vi "5.0.1_LL_Restriction.vi"(6 "Data in":T1, 8 "error in (no error)":errorcluster, 9 "AllControls In":T2, 10 "?":T3, 11 "Message Queue out":T4) -> (0 "error out":errorcluster, 1 "Flow":string, 2 "Data":T3, 3 "Message Queue Out":T4, 4 "Data out":T1)   [LabVIEW 2017]
uses:
  Depends/AMC/subVIs/TypeDefs/amc_Message Queue.ctl
  Depends/AMC/subVIs/TypeDefs/amc_Message.ctl
  Depends/Tools/Keyed Array/Tools_KeyedArray KeyedArray.ctl
  Ctrls/Data.ctl
  Ctrls/AllControls.ctl
  Ctrls/CSV_Data.ctl
  Ctrls/AlarmIndex.ctl
  DIPC 692 Daemon API/typdef/get_parameter.ctl
  DIPC 692 Daemon API/typdef/task_detect_test_point.ctl
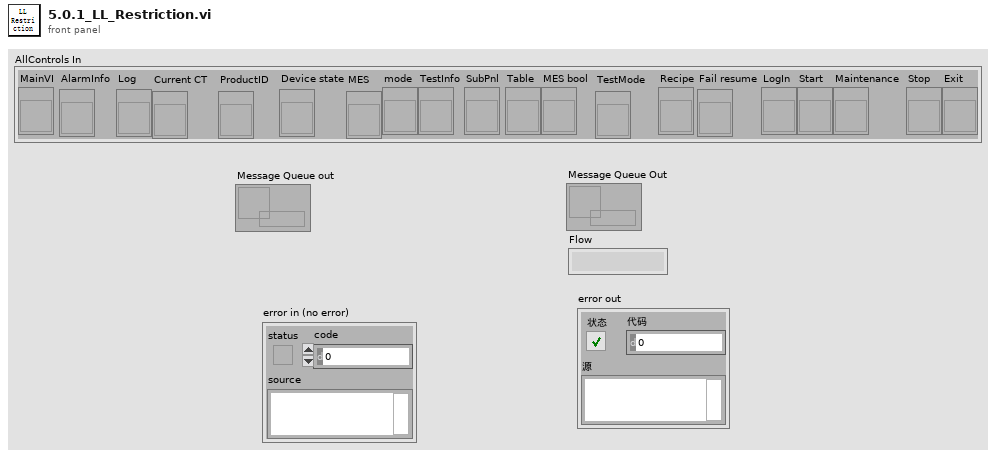
[diagram p1: front panel]
types:
  T1 = typedef "CSV_Data.ctl" = cluster{"Initialisation":cluster{"LMT - Connect UUT (con COM)":string, "LMT - Software Version (rrel)":string, "LMT - Write SKU file (wskuc)":string, "LMT - SKU file name":string, "Connect UUT DDM":string, "Read DDM EOL Timestamp - Mode":string, "Read DDM EOL Timestamp - Timestamp":string, "Read DDM EOL Timestamp - Rig ID":string, "Read DDM EOL Timestamp - Passmark ID":string, "Read DDM EOL Timestamp - Passmark Rev":string, "Software Version before flashing":string, "Read Hardware Serial":string, "UUT DDM SN":string, "Compare DDM SN with MES SN":string, "Backup PCBA Calibration EEPROM Response - CAL":string, "Flash Firmware Version":string, "Check SW Version":string, "Read DDM SW Version after flashing":string, "Set SKU Config":string, "Ready Status":string, "Set Device Mode to EOL":string, "DDM Parameter - Voltage":string, "DDM Parameter - Current":string, "DDM Parameter - Power":string, "DDM Parameter - Speed":string, "DDM Parameter - Pressure":string, "Tester Parameter - Voltage":string, "Tester Parameter - Current":string, "Tester Parameter - Power":string, "Tester Parameter - Ambient Pressure":string, "Tester Parameter - Ambient Temperature":string, "Calculated Parameter - DDM Pressure Corrected":string, "Calculated Parameter - DDM Real Power":string, "Calculated Parameter - Delta V":string}, "BEMF_Calibration":cluster{"Calibration Result - eol_cold_bemf_temp":string, "DDM Ambient Temp":string, "Restriction Plate Diameter":string, "Calibration Result - eol_bemf_mp_cold_coef_a":string, "Calibration Result - eol_bemf_mp_cold_coef_b":string, "Calibration Result - eol_bemf_mp_cold_coef_c":string, "Calibration Result - eol_bemf_lsi_cold_ref_coeffs":string, "Get - Calibration Result - eol_bemf_lsi_speed":string, "Get - Calibration Result - eol_bemf_lsi_integral_0":string, "Calibration Result - eol_bemf_lsi_integral_1":string, "Get - Calibration Result - eol_bemf_lsi_integral_2":string, "Get - Calibration Result - eol_cold_bemf":string, "Get - Calibration Result - eol_cold_bemf_fisf":string, "Finalise Calibration":string, "Compare -Calibration Result - eol_cold_bemf":string, "Compare -Calibration Result - eol_cold_bemf_fisf":string}, "ECO":cluster{"Reset Power Tune":string, "Reset BEMF FISF Calibration":string, "Restriction Plate Diameter":string, "ECO - Stabilisation Time":string, "ECO - DDM Parameter - Voltage":string, "ECO - DDM Parameter - Current":string, "ECO - DDM Parameter - Power":string, "ECO - DDM Parameter - Measured Power":string, "ECO - DDM Parameter - Speed":string, "ECO - DDM Parameter - Pressure":string, "ECO - Tester Parameter - Voltage":string, "ECO - Tester Parameter - Current":string, "ECO - Tester Parameter - Power":string, "ECO - Tester Parameter - Ambient Pressure":string, "ECO - Tester Parameter - Ambient Temperature":string, "ECO - Tester Parameter - Ambient Humidity":string, "ECO - Calculated Parameter - DDM Pressure Corrected":string, "ECO - Calculated Parameter - DDM Real Power":string, "ECO - Calculated Parameter - Delta V":string, "ECO - Calculated Parameter - Flowrate":string, "ECO - Calculated Parameter - Airwatt":string, "ECO - Formula":string, "PT ECO - Power Tune Mode Status":string}, "BOOST":cluster{"Restriction Plate Diameter":string, "BOOST - Stabilisation Time":string, "BOOST - DDM Parameter - Voltage":string, "BOOST - DDM Parameter - Current":string, "BOOST - DDM Parameter - Power":string, "BOOST - DDM Parameter - Measured Power":string, "BOOST - DDM Parameter - Speed":string, "BOOST - DDM Parameter - Pressure":string, "BOOST - Tester Parameter - Voltage":string, "BOOST - Tester Parameter - Current":string, "BOOST - Tester Parameter - Power":string, "BOOST - Tester Parameter - Ambient Pressure":string, "BOOST - Tester Parameter - Ambient Temperature":string, "BOOST - Tester Parameter - Ambient Humidity":string, "BOOST - Calculated Parameter - DDM Pressure Corrected":string, "BOOST - Calculated Parameter - DDM Real Power":string, "BOOST - Calculated Parameter - Delta V":string, "BOOST - Calculated Parameter - Flowrate":string, "BOOST - Calculated Parameter - Airwatt":string, "BOOST - Get AM Presence":string, "Air Muscle Turn Off Status":string, "BOOST - Air Muscle Calculated Parameter - Airwatt B":string, "BOOST - Air Muscle Calculate Airwatt Delta":string, "PT BOOST - Power Tune Mode Status":string, "Finalise Calibration":string, "ECO - Get AW Calibration value":string, "BOOST - Get AW Calibration value":string}, "MAX":cluster{"Restriction Plate Diameter":string, "MAX - Stabilisation Time":string, "Get Average Delta Tmag (LSIdelta_FISFdelta_LSItmag_FISFtmag_IIRtmag)":string, "Get Average Delta Tmag FISF":string, "MAX - DDM Parameter - Voltage":string, "MAX - DDM Parameter - Current":string, "MAX - DDM Parameter - Power":string, "MAX - DDM Parameter - Measured Power":string, "MAX - DDM Parameter - Speed":string, "MAX - DDM Parameter - Pressure":string, "MAX - Tester Parameter - Voltage":string, "MAX - Tester Parameter - Current":string, "MAX - Tester Parameter - Power":string, "MAX - Tester Parameter - Ambient Pressure":string, "MAX - Tester Parameter - Ambient Temperature":string, "MAX - Tester Parameter - Ambient Humidity":string, "MAX - Calculated Parameter - DDM Pressure Corrected":string, "MAX - Calculated Parameter - DDM Real Power":string, "MAX - Calculated Parameter - Delta V":string, "MAX - Calculated Parameter - Flowrate":string, "MAX - Calculated Parameter - Airwatt":string, "MAX_FISF_Check_Average_Delta_Tmag":string, "MAX - FISF - BEMF Finetune Result":string, "MAX tune - Delta P1":string, "MAX tune - Calculated Parameter - Airwatt":string, "Calculate Delta Airwatts - MAX finetune - Delta P2":string, "MAX finetune - DDM Parameter - Voltage":string, "MAX finetune - DDM Parameter - Current":string, "MAX finetune - DDM Parameter - Power":string, "MAX finetune - DDM Parameter - Measured Power":string, "MAX finetune - DDM Parameter - Speed":string, "MAX finetune - DDM Parameter - Pressure":string, "MAX finetune - Tester Parameter - Voltage":string, "MAX finetune - Tester Parameter - Current":string, "MAX finetune - Tester Parameter - Power":string, "MAX finetune - Tester Parameter - Ambient Pressure":string, "MAX finetune - Tester Parameter - Ambient Temperature":string, "MAX finetune - Tester Parameter - Ambient Humidity":string, "MAX finetune - Calculated Parameter - DDM Pressure Corrected":string, "MAX finetune - Calculated Parameter - DDM Real Power":string, "MAX finetune - Calculated Parameter - Delta V":string, "MAX finetune - Calculated Parameter - Flowrate":string, "MAX finetune - Calculated Parameter - Airwatt":string, "Check Derate Result":string, "Delta Tmag FISF":string, "Get Hot BEMF Result":string, "Calculate delta Pressure":string, "Finalise Calibration":string, "Calculate & Check Delta BEMF":string, "Delta P Airwatts Value":string}, "LL":cluster{"DDM Ambient Temp":string, "Restriction Plate Diameter":string, "LL - DDM Parameter - Voltage":string, "LL - DDM Parameter - Current":string, "LL - DDM Parameter - Power":string, "LL - DDM Parameter - Measured Power":string, "LL - DDM Parameter - Speed":string, "LL - DDM Parameter - Pressure":string, "LL - Tester Parameter - Voltage":string, "LL - Tester Parameter - Current":string, "LL - Tester Parameter - Power":string, "LL - DDM Real Power":string, "LL - Calibrate Task Detect LL":string}, "HL":cluster{"HL - DDM Parameter - Voltage":string, "HL - DDM Parameter - Current":string, "HL - DDM Parameter - Power":string, "HL - DDM Parameter - Measured Power":string, "HL - DDM Parameter - Speed":string, "HL - DDM Parameter - Pressure":string, "HL - Tester Parameter - Voltage":string, "HL - Tester Parameter - Current":string, "HL - Tester Parameter - Power":string, "HL - DDM Real Power":string, "HL - Calibrate Task Detect HL":string}, "LH":cluster{"Restriction Plate Diameter":string, "LH - DDM Parameter - Voltage":string, "LH - DDM Parameter - Current":string, "LH - DDM Parameter - Power":string, "LH - DDM Parameter - Measured Power":string, "LH - DDM Parameter - Speed":string, "LH - DDM Parameter - Pressure":string, "LH - Tester Parameter - Voltage":string, "LH - Tester Parameter - Current":string, "LH - Tester Parameter - Power":string, "LH - DDM Real Power":string, "LH - Calibrate Task Detect LH":string}, "HH":cluster{"HH - DDM Parameter - Voltage":string, "HH - DDM Parameter - Current":string, "HH - DDM Parameter - Power":string, "HH - DDM Parameter - Measured Power":string, "HH - DDM Parameter - Speed":string, "HH - DDM Parameter - Pressure":string, "HH - Tester Parameter - Voltage":string, "HH - Tester Parameter - Current":string, "HH - Tester Parameter - Power":string, "HH - DDM Real Power":string, "HH - Calibrate Task Detect HH":string}, "Inlet Blockage Calibration":cluster{"Inlet Blockage Calibration - DDM Parameter - Voltage":string, "Inlet Blockage Calibration - DDM Parameter - Current":string, "Inlet Blockage Calibration - DDM Parameter - Power":string, "Inlet Blockage Calibration - DDM Parameter - Measured Power":string, "Inlet Blockage Calibration - DDM Parameter - Speed":string, "Inlet Blockage Calibration - DDM Parameter - Pressure":string, "Inlet Blockage Calibration - Tester Parameter - Voltage":string, "Inlet Blockage Calibration - Tester Parameter - Current":string, "Inlet Blockage Calibration - Tester Parameter - Power":string, "Inlet Blockage Calibration - DDM Real Power":string, "Calibration Inlet Blockage_E":string, "Finalise Calibration":string, "Get Task Detect LL":string, "Get Task Detect HL":string, "Get Task Detect LH":string, "Get Task Detect HH":string, "Calibration Inlet Blockage":string, "Calibration eol cold bemf temp":string}, "GOOD":cluster{"GOOD UNIT - Clear EEPROM Error Log":string, "GOOD UNIT - Write Product Timestamp - Mode":string, "GOOD UNIT - Write Product Timestamp - Timestamp":string, "GOOD UNIT - Write Product Timestamp - Rig ID":string, "GOOD UNIT - Write Product Timestamp - Passmark ID":string, "GOOD UNIT - Write Product Timestamp - Passmark Rev":string, "GOOD UNIT - Set Device Mode to PROD":string, "GOOD UNIT - Backup PCBA Calibration EEPROM Response":string, "GOOD UNIT - Check Security Bit":string, "GOOD UNIT - Set Calibration Lock":string, "GOOD UNIT - Get_Calibration_Lock":string, "GOOD UNIT - Disconnect UUT":string}, "NG":cluster{"NG UNIT - Read NVM Error":string, "NG UNIT - Set Device Mode to FCT":string, "NG UNIT - Backup PCBA Calibration EEPROM Response - CAL":string, "NG UNIT - Backup PCBA Calibration EEPROM Response - ERROR":string, "NG UNIT - Backup PCBA Calibration EEPROM Response - USAGE":string, "NG UNIT - Disconnect UUT":string}, "SN":string, "Table":string[][], "Count":cluster{"Total":i32, "OK":i32, "NG":i32, "Yield":dbl}, "Start Time":timestamp, "daemon reference":refnum<k5>, "CT":dbl, "Config":string[][], "OK/NG":bool, "Station ID":string, "MES DDM SN":string, "MES PCBA SN":string, "Retest":string, "Lux":string, "Initialisation_Status":cluster{"LMT - Connect UUT (con COM)":string, "LMT - Software Version (rrel)":string, "LMT - Write SKU file (wskuc)":string, "LMT - SKU file name":string, "Connect UUT DDM":string, "Read DDM EOL Timestamp - Mode":string, "Read DDM EOL Timestamp - Timestamp":string, "Read DDM EOL Timestamp - Rig ID":string, "Read DDM EOL Timestamp - Passmark ID":string, "Read DDM EOL Timestamp - Passmark Rev":string, "Software Version before flashing":string, "Read Hardware Serial":string, "UUT DDM SN":string, "Compare DDM SN with MES SN":string, "Backup PCBA Calibration EEPROM Response - CAL":string, "Flash Firmware Version":string, "Check SW Version":string, "Read DDM SW Version after flashing":string, "Set SKU Config":string, "Ready Status":string, "Set Device Mode to EOL":string, "DDM Parameter - Voltage":string, "DDM Parameter - Current":string, "DDM Parameter - Power":string, "DDM Parameter - Speed":string, "DDM Parameter - Pressure":string, "Tester Parameter - Voltage":string, "Tester Parameter - Current":string, "Tester Parameter - Power":string, "Tester Parameter - Ambient Pressure":string, "Tester Parameter - Ambient Temperature":string, "Calculated Parameter - DDM Pressure Corrected":string, "Calculated Parameter - DDM Real Power":string, "Calculated Parameter - Delta V":string}, "BEMF_Calibration_Status":cluster{"Calibration Result - eol_cold_bemf_temp":string, "DDM Ambient Temp":string, "Restriction Plate Diameter":string, "Calibration Result - eol_bemf_mp_cold_coef_a":string, "Calibration Result - eol_bemf_mp_cold_coef_b":string, "Calibration Result - eol_bemf_mp_cold_coef_c":string, "Calibration Result - eol_bemf_lsi_cold_ref_coeffs":string, "Get - Calibration Result - eol_bemf_lsi_speed":string, "Get - Calibration Result - eol_bemf_lsi_integral_0":string, "Calibration Result - eol_bemf_lsi_integral_1":string, "Get - Calibration Result - eol_bemf_lsi_integral_2":string, "Get - Calibration Result - eol_cold_bemf":string, "Get - Calibration Result - eol_cold_bemf_fisf":string, "Finalise Calibration":string, "Compare -Calibration Result - eol_cold_bemf":string, "Compare -Calibration Result - eol_cold_bemf_fisf":string}, "ECO_Status":cluster{"Reset Power Tune":string, "Reset BEMF FISF Calibration":string, "Restriction Plate Diameter":string, "ECO - Stabilisation Time":string, "ECO - DDM Parameter - Voltage":string, "ECO - DDM Parameter - Current":string, "ECO - DDM Parameter - Power":string, "ECO - DDM Parameter - Measured Power":string, "ECO - DDM Parameter - Speed":string, "ECO - DDM Parameter - Pressure":string, "ECO - Tester Parameter - Voltage":string, "ECO - Tester Parameter - Current":string, "ECO - Tester Parameter - Power":string, "ECO - Tester Parameter - Ambient Pressure":string, "ECO - Tester Parameter - Ambient Temperature":string, "ECO - Tester Parameter - Ambient Humidity":string, "ECO - Calculated Parameter - DDM Pressure Corrected":string, "ECO - Calculated Parameter - DDM Real Power":string, "ECO - Calculated Parameter - Delta V":string, "ECO - Calculated Parameter - Flowrate":string, "ECO - Calculated Parameter - Airwatt":string, "ECO - Formula":string, "PT ECO - Power Tune Mode Status":string}, "BOOST_Status":cluster{"Restriction Plate Diameter":string, "BOOST - Stabilisation Time":string, "BOOST - DDM Parameter - Voltage":string, "BOOST - DDM Parameter - Current":string, "BOOST - DDM Parameter - Power":string, "BOOST - DDM Parameter - Measured Power":string, "BOOST - DDM Parameter - Speed":string, "BOOST - DDM Parameter - Pressure":string, "BOOST - Tester Parameter - Voltage":string, "BOOST - Tester Parameter - Current":string, "BOOST - Tester Parameter - Power":string, "BOOST - Tester Parameter - Ambient Pressure":string, "BOOST - Tester Parameter - Ambient Temperature":string, "BOOST - Tester Parameter - Ambient Humidity":string, "BOOST - Calculated Parameter - DDM Pressure Corrected":string, "BOOST - Calculated Parameter - DDM Real Power":string, "BOOST - Calculated Parameter - Delta V":string, "BOOST - Calculated Parameter - Flowrate":string, "BOOST - Calculated Parameter - Airwatt":string, "BOOST - Get AM Presence":string, "Air Muscle Turn Off Status":string, "BOOST - Air Muscle Calculated Parameter - Airwatt B":string, "BOOST - Air Muscle Calculate Airwatt Delta":string, "PT BOOST - Power Tune Mode Status":string, "Finalise Calibration":string, "ECO - Get AW Calibration value":string, "BOOST - Get AW Calibration value":string}, "MAX_Status":cluster{"Restriction Plate Diameter":string, "MAX - Stabilisation Time":string, "Get Average Delta Tmag (LSIdelta_FISFdelta_LSItmag_FISFtmag_IIRtmag)":string, "Get Average Delta Tmag FISF":string, "MAX - DDM Parameter - Voltage":string, "MAX - DDM Parameter - Current":string, "MAX - DDM Parameter - Power":string, "MAX - DDM Parameter - Measured Power":string, "MAX - DDM Parameter - Speed":string, "MAX - DDM Parameter - Pressure":string, "MAX - Tester Parameter - Voltage":string, "MAX - Tester Parameter - Current":string, "MAX - Tester Parameter - Power":string, "MAX - Tester Parameter - Ambient Pressure":string, "MAX - Tester Parameter - Ambient Temperature":string, "MAX - Tester Parameter - Ambient Humidity":string, "MAX - Calculated Parameter - DDM Pressure Corrected":string, "MAX - Calculated Parameter - DDM Real Power":string, "MAX - Calculated Parameter - Delta V":string, "MAX - Calculated Parameter - Flowrate":string, "MAX - Calculated Parameter - Airwatt":string, "MAX_FISF_Check_Average_Delta_Tmag":string, "MAX - FISF - BEMF Finetune Result":string, "MAX tune - Delta P1":string, "MAX tune - Calculated Parameter - Airwatt":string, "Calculate Delta Airwatts - MAX finetune - Delta P2":string, "MAX finetune - DDM Parameter - Voltage":string, "MAX finetune - DDM Parameter - Current":string, "MAX finetune - DDM Parameter - Power":string, "MAX finetune - DDM Parameter - Measured Power":string, "MAX finetune - DDM Parameter - Speed":string, "MAX finetune - DDM Parameter - Pressure":string, "MAX finetune - Tester Parameter - Voltage":string, "MAX finetune - Tester Parameter - Current":string, "MAX finetune - Tester Parameter - Power":string, "MAX finetune - Tester Parameter - Ambient Pressure":string, "MAX finetune - Tester Parameter - Ambient Temperature":string, "MAX finetune - Tester Parameter - Ambient Humidity":string, "MAX finetune - Calculated Parameter - DDM Pressure Corrected":string, "MAX finetune - Calculated Parameter - DDM Real Power":string, "MAX finetune - Calculated Parameter - Delta V":string, "MAX finetune - Calculated Parameter - Flowrate":string, "MAX finetune - Calculated Parameter - Airwatt":string, "Check Derate Result":string, "Delta Tmag FISF":string, "Get Hot BEMF Result":string, "Calculate delta Pressure":string, "Finalise Calibration":string, "Calculate & Check Delta BEMF":string, "Delta P Airwatts Value":string}, "LL_Status":cluster{"DDM Ambient Temp":string, "Restriction Plate Diameter":string, "LL - DDM Parameter - Voltage":string, "LL - DDM Parameter - Current":string, "LL - DDM Parameter - Power":string, "LL - DDM Parameter - Measured Power":string, "LL - DDM Parameter - Speed":string, "LL - DDM Parameter - Pressure":string, "LL - Tester Parameter - Voltage":string, "LL - Tester Parameter - Current":string, "LL - Tester Parameter - Power":string, "LL - DDM Real Power":string, "LL - Calibrate Task Detect LL":string}, "HL_Status":cluster{"HL - DDM Parameter - Voltage":string, "HL - DDM Parameter - Current":string, "HL - DDM Parameter - Power":string, "HL - DDM Parameter - Measured Power":string, "HL - DDM Parameter - Speed":string, "HL - DDM Parameter - Pressure":string, "HL - Tester Parameter - Voltage":string, "HL - Tester Parameter - Current":string, "HL - Tester Parameter - Power":string, "HL - DDM Real Power":string, "HL - Calibrate Task Detect HL":string}, "LH_Status":cluster{"Restriction Plate Diameter":string, "LH - DDM Parameter - Voltage":string, "LH - DDM Parameter - Current":string, "LH - DDM Parameter - Power":string, "LH - DDM Parameter - Measured Power":string, "LH - DDM Parameter - Speed":string, "LH - DDM Parameter - Pressure":string, "LH - Tester Parameter - Voltage":string, "LH - Tester Parameter - Current":string, "LH - Tester Parameter - Power":string, "LH - DDM Real Power":string, "LH - Calibrate Task Detect LH":string}, "HH_Status":cluster{"HH - DDM Parameter - Voltage":string, "HH - DDM Parameter - Current":string, "HH - DDM Parameter - Power":string, "HH - DDM Parameter - Measured Power":string, "HH - DDM Parameter - Speed":string, "HH - DDM Parameter - Pressure":string, "HH - Tester Parameter - Voltage":string, "HH - Tester Parameter - Current":string, "HH - Tester Parameter - Power":string, "HH - DDM Real Power":string, "HH - Calibrate Task Detect HH":string}, "Inlet Blockage Calibration_Status":cluster{"Inlet Blockage Calibration - DDM Parameter - Voltage":string, "Inlet Blockage Calibration - DDM Parameter - Current":string, "Inlet Blockage Calibration - DDM Parameter - Power":string, "Inlet Blockage Calibration - DDM Parameter - Measured Power":string, "Inlet Blockage Calibration - DDM Parameter - Speed":string, "Inlet Blockage Calibration - DDM Parameter - Pressure":string, "Inlet Blockage Calibration - Tester Parameter - Voltage":string, "Inlet Blockage Calibration - Tester Parameter - Current":string, "Inlet Blockage Calibration - Tester Parameter - Power":string, "Inlet Blockage Calibration - DDM Real Power":string, "Calibration Inlet Blockage_E":string, "Finalise Calibration":string, "Get Task Detect LL":string, "Get Task Detect HL":string, "Get Task Detect LH":string, "Get Task Detect HH":string, "Calibration Inlet Blockage":string, "Calibration eol cold bemf temp":string}, "GOOD_Status":cluster{"GOOD UNIT - Clear EEPROM Error Log":string, "GOOD UNIT - Write Product Timestamp - Mode":string, "GOOD UNIT - Write Product Timestamp - Timestamp":string, "GOOD UNIT - Write Product Timestamp - Rig ID":string, "GOOD UNIT - Write Product Timestamp - Passmark ID":string, "GOOD UNIT - Write Product Timestamp - Passmark Rev":string, "GOOD UNIT - Set Device Mode to PROD":string, "GOOD UNIT - Backup PCBA Calibration EEPROM Response":string, "GOOD UNIT - Check Security Bit":string, "GOOD UNIT - Set Calibration Lock":string, "GOOD UNIT - Get_Calibration_Lock":string, "GOOD UNIT - Disconnect UUT":string}, "NG_Status":cluster{"NG UNIT - Read NVM Error":string, "NG UNIT - Set Device Mode to FCT":string, "NG UNIT - Backup PCBA Calibration EEPROM Response - CAL":string, "NG UNIT - Backup PCBA Calibration EEPROM Response - ERROR":string, "NG UNIT - Backup PCBA Calibration EEPROM Response - USAGE":string, "NG UNIT - Disconnect UUT":string}, "SKU":string, "Plate_Diameter":string, "Alarm":string}
  T2 = typedef "AllControls.ctl" = cluster{"MainVI":refnum<vi>, "AlarmInfo":refnum<vi>, "Log":refnum<vi>, "Current CT":refnum<vi>, "ProductID":refnum<vi>, "Device state":refnum<vi>, "MES":refnum<vi>, "mode":refnum<vi>, "TestInfo":refnum<vi>, "SubPnl":refnum<vi>, "Table":refnum<vi>, "MES bool":refnum<vi>, "TestMode":refnum<vi>, "Recipe":refnum<vi>, "Fail resume":refnum<vi>, "LogIn":refnum<vi>, "Start":refnum<vi>, "Maintenance":refnum<vi>, "Stop":refnum<vi>, "Exit":refnum<vi>}
  T3 = typedef "Data.ctl" = cluster{"Initialisation":cluster{"DDM_Parameter":dbl[], "DDM_Parameter_status":bool[], "Get_Tester_Parameter":dbl[], "Get_Tester_Parameter_status":bool[], "Cal_Tester_Parameter":dbl[], "Cal_Tester_Parameter_status":bool[], "sw_version_before_status":bool, "sw_version_after_status":bool, "Set_SKU_Config_With_LMT_status":bool, "FCT_timestamp_status":bool, "LMT_Connect_to_UUT_status":bool}, "BEMF_Calibration":cluster{"Read_ambient_temperature":dbl, "Calibration_Vaule":dbl[], "Calibration_Vaule _B":dbl[], "Calibration_Vaule_status":bool[], "Calibration_Vaule_B_status":bool[]}, "ECO":cluster{"DDM_Parameter":dbl[], "DDM_Parameter_status":bool[], "Get_Tester_Parameter":dbl[], "Get_Tester_Parameter_status":bool[], "Cal_Tester_Parameter":dbl[], "Cal_Tester_Parameter_status":bool[], "DDM_Parameter_after_power_tune":dbl[], "Get_Tester_Parameter_after_power_tune":dbl[], "Cal_Tester_Parameter_after_power_tune":dbl[], "Cal_Tester_Parameter_after_power_tune_status":bool[], "Delta_P":dbl}, "BOOST":cluster{"DDM_Parameter":dbl[], "DDM_Parameter_status":bool[], "Get_Tester_Parameter":dbl[], "Get_Tester_Parameter_status":bool[], "Cal_Tester_Parameter":dbl[], "Cal_Tester_Parameter_status":bool[], "DDM_Parameter_after_power_tune":dbl[], "Get_Tester_Parameter_after_power_tune":dbl[], "Cal_Tester_Parameter_after_power_tune":dbl[], "Cal_Tester_Parameter_after_power_tune_status":bool[], "airwatts_am_off":dbl, "AW_Delta_(AM_on_and_off)":dbl, "AW_Delta_(AM_on_and_off)_Status":bool, "Delta_P":dbl}, "MAX":cluster{"Average_Tmag_Data":cluster{"LSI Delta in degC":dbl, "FISF Delta in degc":dbl, "LSI Tmag in degC":dbl, "Fisf Tmag in degC":dbl, "IIR Tmag in degC":dbl}, "DDM_Parameter":dbl[], "DDM_Parameter_status":bool[], "Get_Tester_Parameter":dbl[], "Get_Tester_Parameter_status":bool[], "Cal_Tester_Parameter":dbl[], "BEMF_Finetune":cluster{"eol_bemf_mp_cold_coef_c":dbl, "eol_cold_bemf_fisf_offset":dbl}, "AW_Tune":cluster{"delta_P1":dbl, "delta_P_Setting":dbl}, "DDM_Parameter_after_Airwatts_Tune":dbl[], "Get_Tester_Parameter_after_Airwatts_Tune":dbl[], "Cal_Tester_Parameter_after_Airwatts_Tune":dbl[], "DDM_Parameter_after_Airwatts_Finetune":dbl[], "Get_Tester_Parameter_after_Airwatts_Finetune":dbl[], "Cal_Tester_Parameter_after_Airwatts_Finetune":dbl[], "AW_Finetune":cluster{"delta_P2":dbl, "delta_P_Setting":dbl}, "Delta_Tmag_after_tune":cluster{"LSI Delta in degC":dbl, "FISF Delta in degc":dbl, "LSI Tmag in degC":dbl, "Fisf Tmag in degC":dbl, "IIR Tmag in degC":dbl}, "Hot Bemf in mV":dbl, "DDM_Pressure":dbl, "Delta_Pressure":dbl, " Cold Bemf in mV":dbl, " delta Bemf":dbl, " delta p":dbl, "Delta_Pressure_status":bool, " delta Bemf_status":bool, "LSI Delta in degC_status":bool, "FISF Delta in degc_status":bool, "Max_check_derate_status_status":bool, "Average_All_data":dbl[][], "Average_Tmag_Data_status":bool[], "Average_Tmag_Data_after_tune_status":bool[], "Cal_Tester_Parameter_status":bool[], "Cal_Tester_Parameter_status_after_Airwatts_Tune":bool[], "Cal_Tester_Parameter_status_after_Airwatts_FineTune":bool[]}, "Task_Detect_Calib":cluster{"LL":cluster{"DDM_Parameter":dbl[], "DDM_Parameter_status":bool[], "Get_Tester_Parameter":dbl[], "Get_Tester_Parameter_status":bool[], "Set_task_detect_A":dbl, "Set_task_detect_A_Status":bool}, "HL":cluster{"DDM_Parameter":dbl[], "DDM_Parameter_status":bool[], "Get_Tester_Parameter":dbl[], "Get_Tester_Parameter_status":bool[], "Set_task_detect_B":dbl, "Set_task_detect_B_Status":bool}, "LH":cluster{"DDM_Parameter":dbl[], "DDM_Parameter_status":bool[], "Get_Tester_Parameter":dbl[], "Get_Tester_Parameter_status":bool[], "Set_task_detect_C":dbl, "Set_task_detect_C_Status":bool}, "HH":cluster{"DDM_Parameter":dbl[], "DDM_Parameter_status":bool[], "Get_Tester_Parameter":dbl[], "Get_Tester_Parameter_status":bool[], "Set_task_detect_D":dbl, "Read_and_check_calibration_Status":bool[], "Set_task_detect_D_Status":bool}, "Get_eol_inlet_blockage_E":dbl, "Calib_vaule":cluster{"Get_task_detect_LL":dbl, "Get_task_detect_HL":dbl, "Get_task_detect_LH":dbl, "Get_task_detect_HH":dbl, "eol_inlet_blockage":dbl, "eol_code_bemf_temp":dbl}, "calibrated temp":dbl, "Inlet_Blockage_Calibration":cluster{"DDM_Parameter":dbl[], "DDM_Parameter_status":bool[], "Get_Tester_Parameter":dbl[], "Get_Tester_Parameter_status":bool[]}, "Get_eol_inlet_blockage_E_Status":bool}, "good":cluster{"Write_Product_TS":cluster{"TIMESTAMP":i64, "RIG_ID":i64, "PASSMARK_ID":i64, "PASSMARK_REV":i64}, "Read_Product_TS":cluster{"TIMESTAMP":i64, "RIG_ID":i64, "PASSMARK_ID":i64, "PASSMARK_REV":i64}, "Good_Check_Secuity_Bit_Stauts":bool}}
  T4 = typedef "amc_Message Queue.ctl" = refnum<queue>
  T5 = typedef "HD Config.ctl" = cluster{" PC":cluster{"PC Address":u8[], "PC Port":i32}, "FCO":cluster{"COM":refnum<visa-resource-name>, "Baudrate":u32}, "DC Power ":cluster{"COM":refnum<visa-resource-name>, "Baudrate":u32}, "PW3336":cluster{"COM":refnum<visa-resource-name>, "Baudrate":u32}, "Lefoo":cluster{"COM":refnum<visa-resource-name>, "Baudrate":u32}, "Tempt&Hum":cluster{"COM":refnum<visa-resource-name>, "Baudrate":u32}, "DIPC":cluster{"COM":refnum<visa-resource-name>}, "Daemon":cluster{"IP Address":string, "Port":u16, "Retry":u16}, "NFC":cluster{"COM":refnum<visa-resource-name>, "Baudrate":u32}, "Fail_resume_mode":bool, "GRR":bool}
  T6 = typedef "AlarmIndex.ctl" = enum16{"E-Stop", "Safety light grid", "UUT Sealing Cylinder HomePoint", "UUT Sealing Cylinder WorkPoint", "Orifice fixed Cylinder L HomePoint", "Orifice fixed Cylinder L WorkPoint", "Orifice fixed Cylinder R HomePoint", "Orifice fixed Cylinder R WorkPoint", "UUT Cylinder HomePoint", "UUT Cylinder WorkPoint", "Carrier fixed Cylinder L HomePoint", "Carrier fixed Cylinder L WorkPoint", "Carrier fixed Cylinder R HomePoint", "Carrier fixed Cylinder R WorkPoint", "Probe Cylinder HomePoint", "Probe Cylinder WorkPoint", "Motor Error", "Test Error"}
  T7 = typedef "get_parameter.ctl" = string
  T8 = typedef "task_detect_test_point.ctl" = enum16{"LL", "HL", "LH", "HH"}
  T9 = typedef "Position Config.ctl" = cluster{"Black":i32, "White":i32, "Black1":i32, "White1":i32}
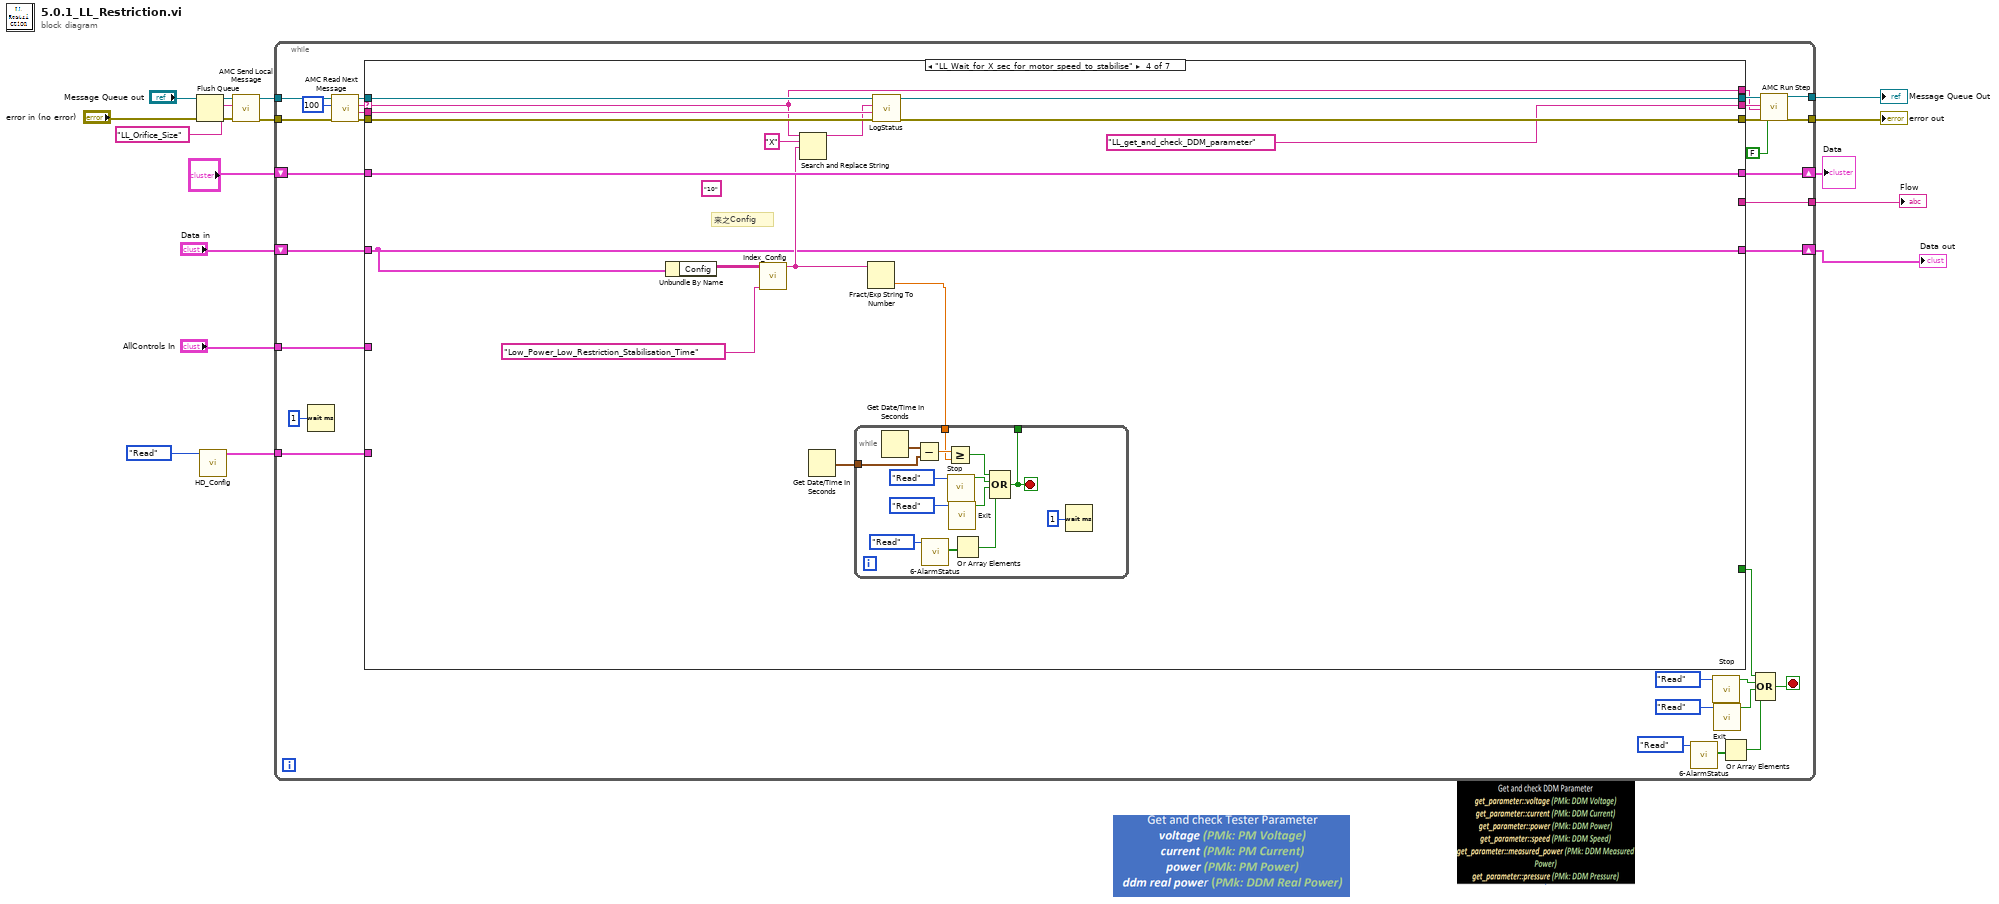
[diagram p0: block diagram]
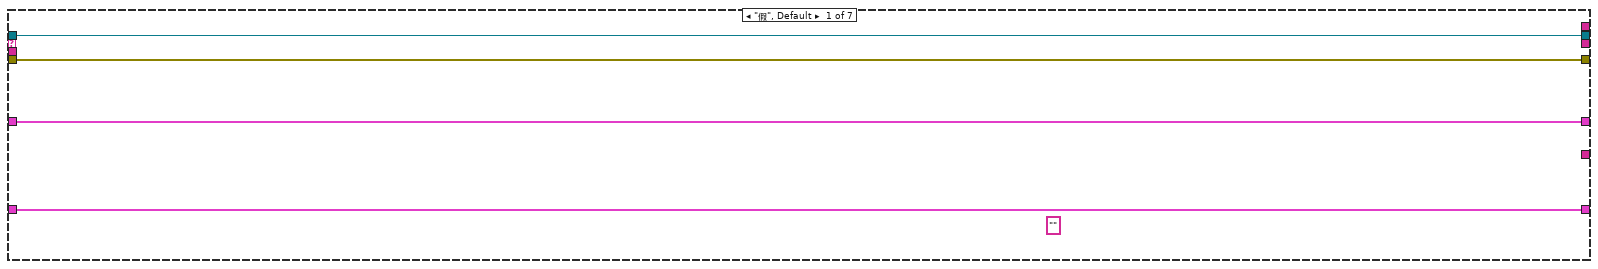
[diagram p2: hidden frame]
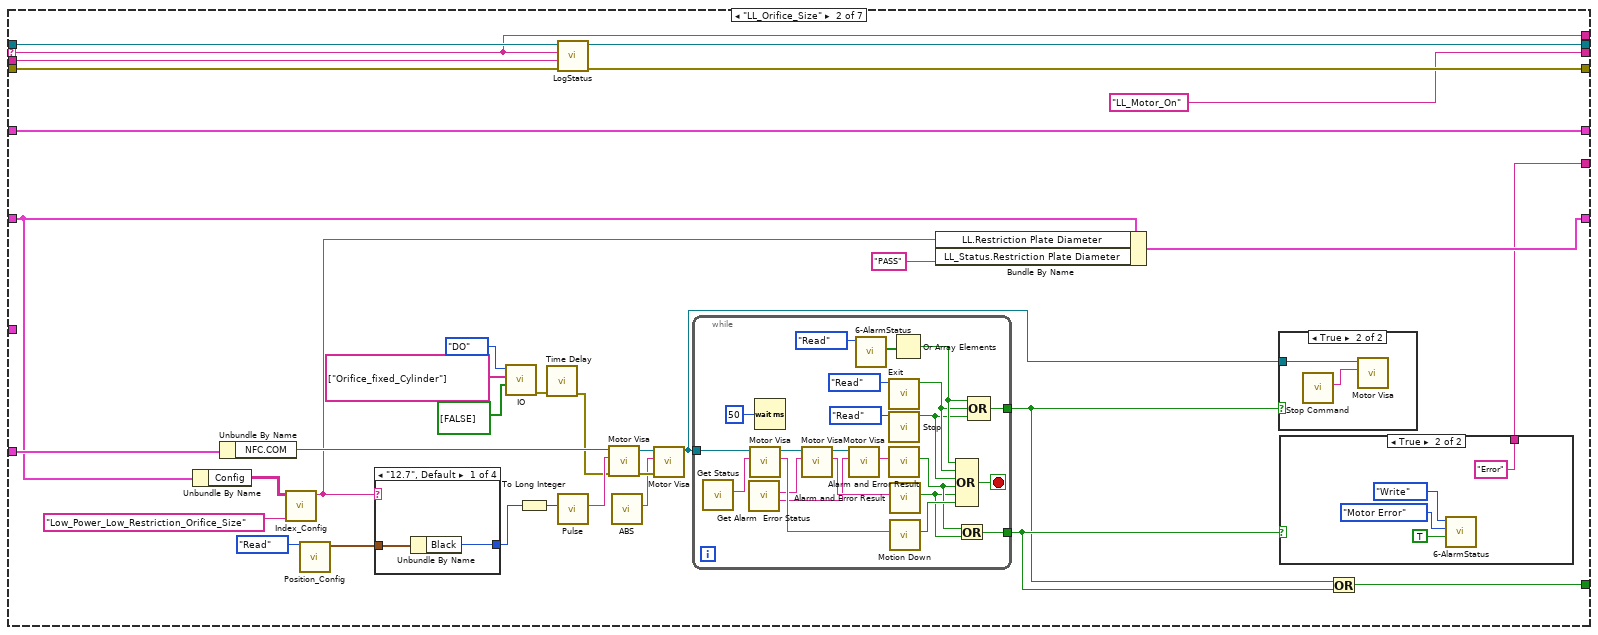
[diagram p3: hidden frame]
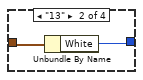
[diagram p5: hidden frame]
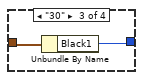
[diagram p6: hidden frame]
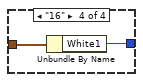
[diagram p7: hidden frame]
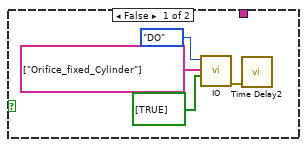
[diagram p8: hidden frame]
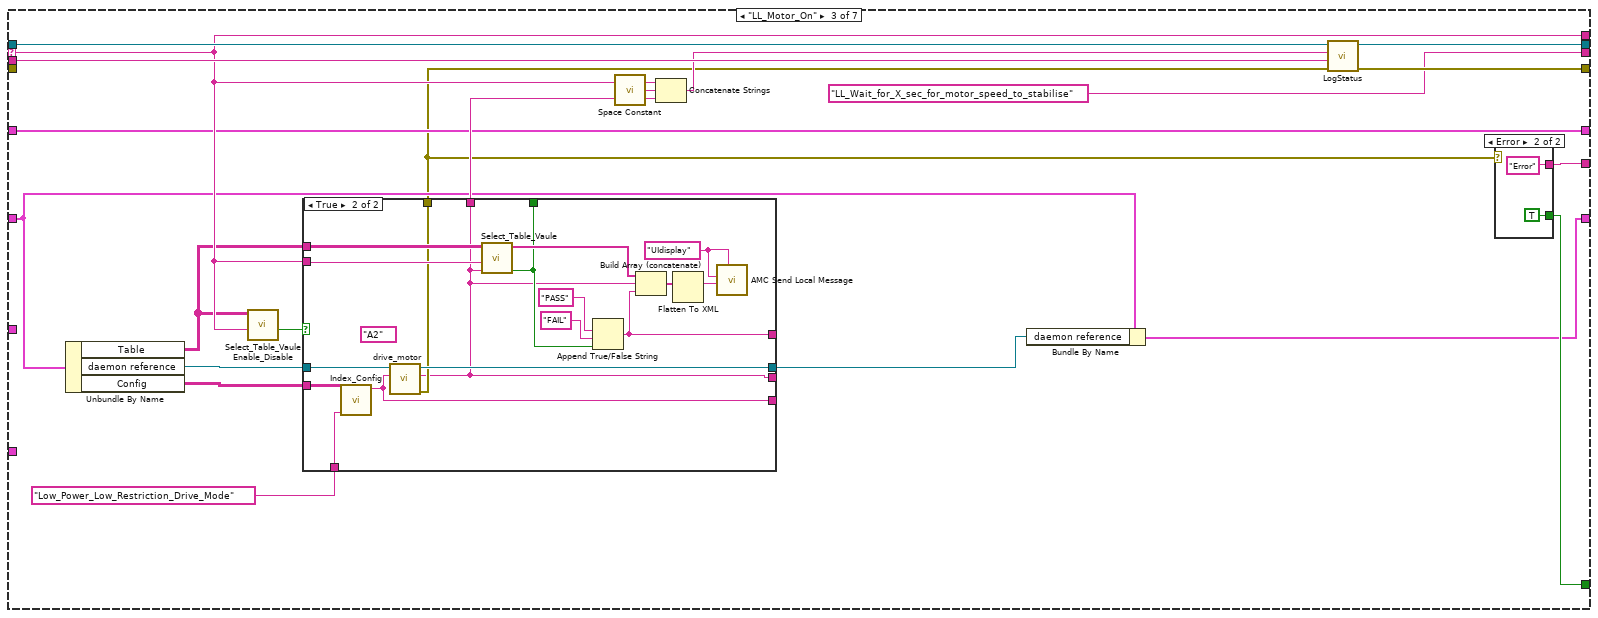
[diagram p9: hidden frame]
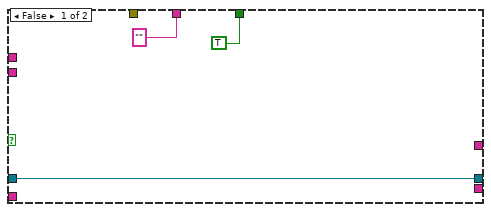
[diagram p11: hidden frame]
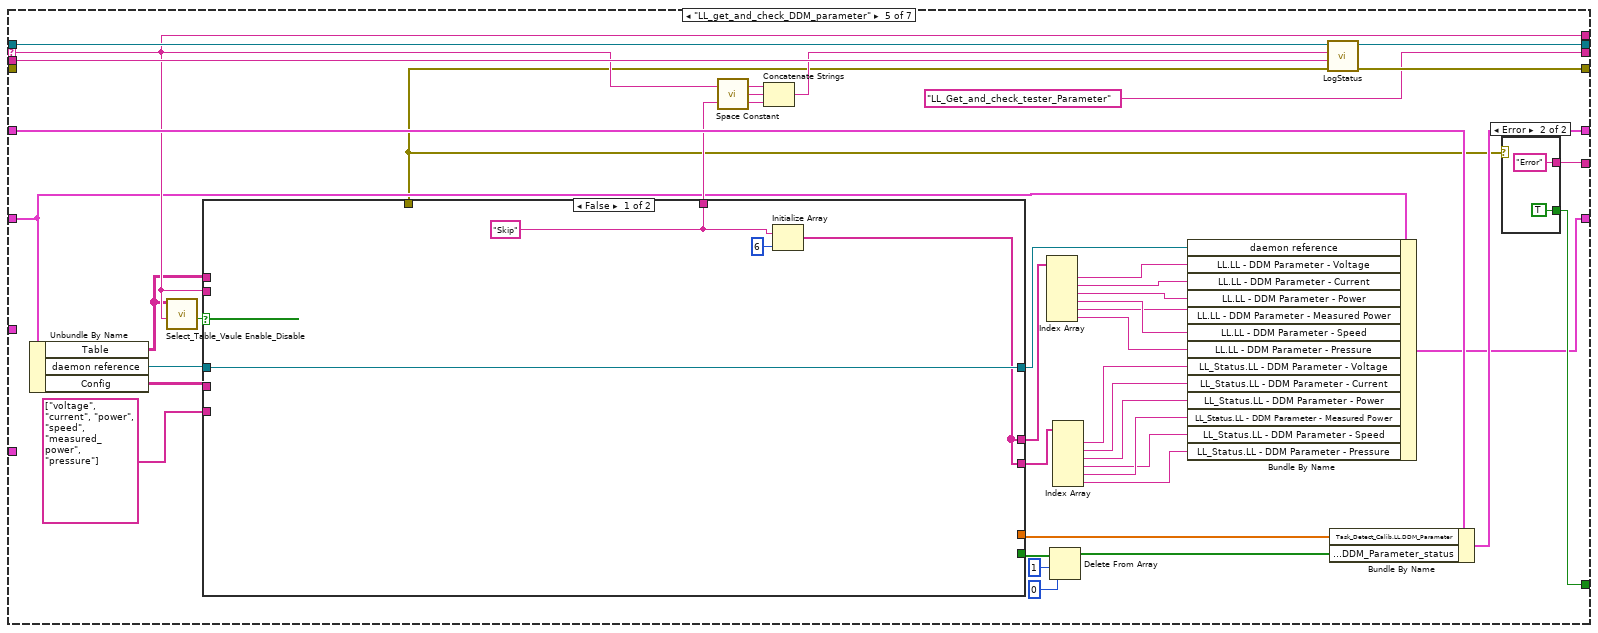
[diagram p12: hidden frame]
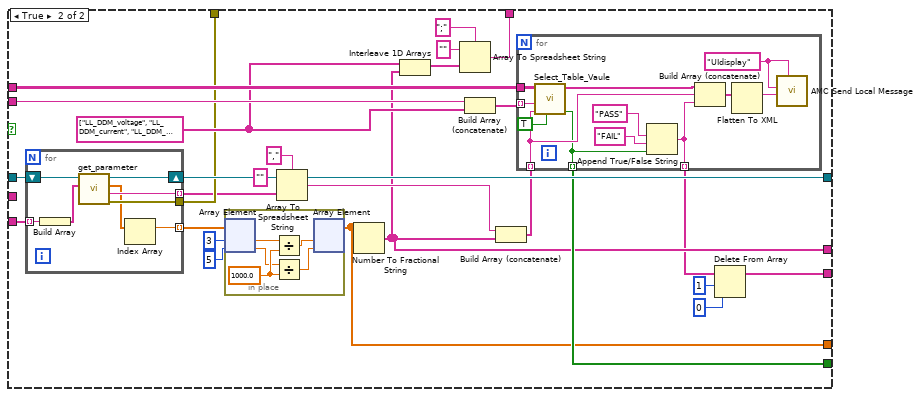
[diagram p14: hidden frame]
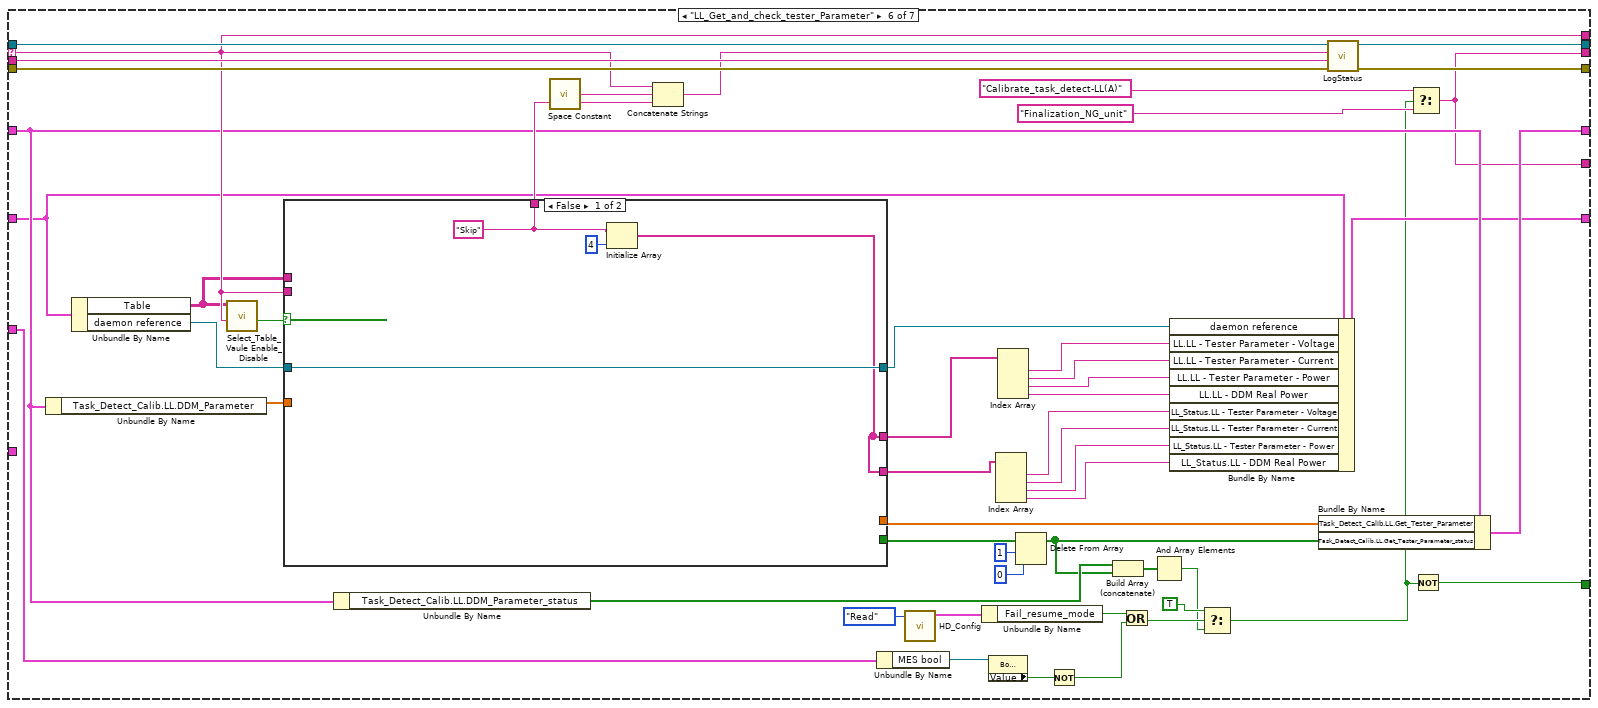
[diagram p15: hidden frame]
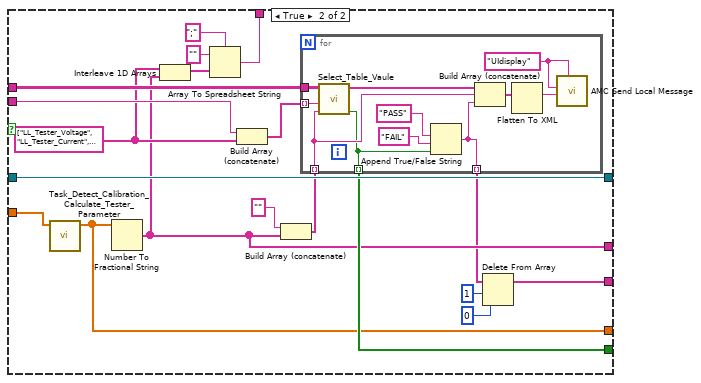
[diagram p16: hidden frame]
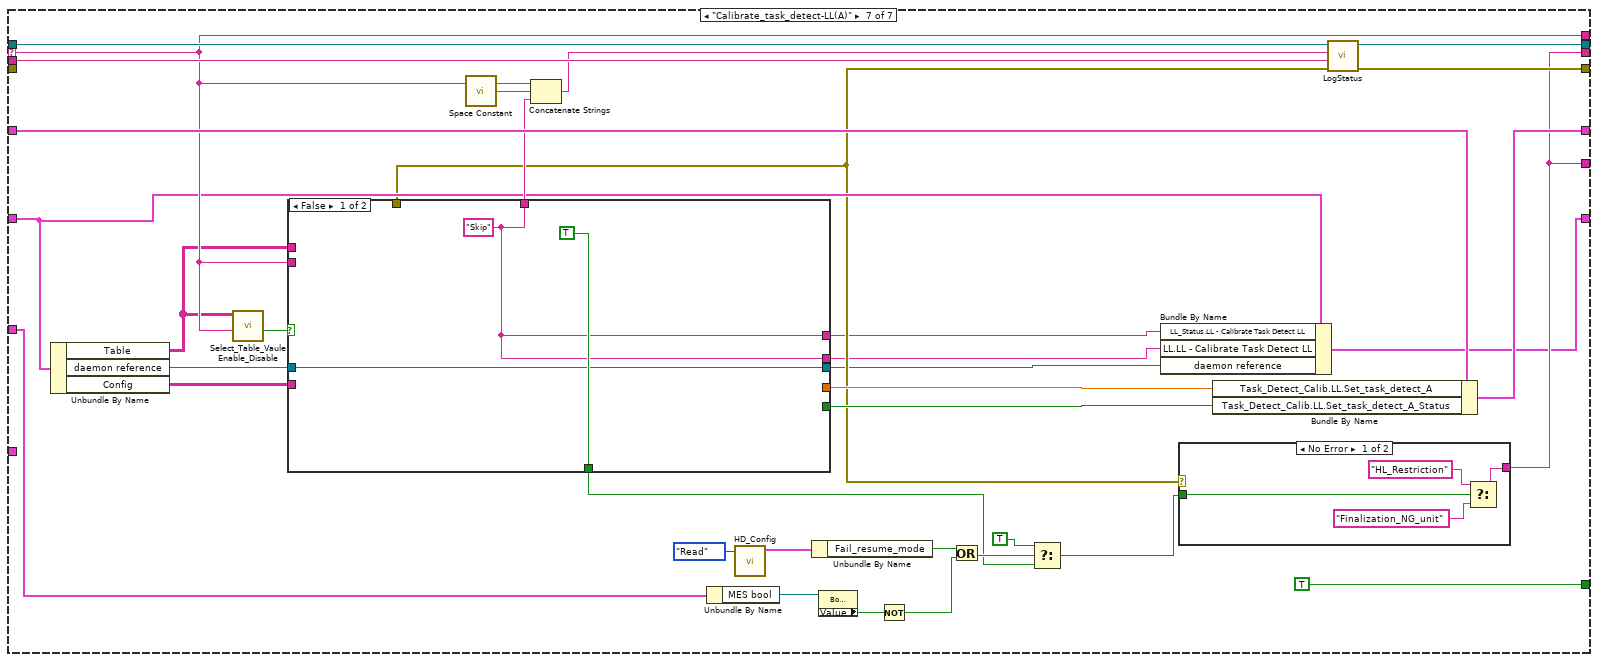
[diagram p17: hidden frame]
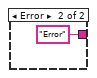
[diagram p18: hidden frame]
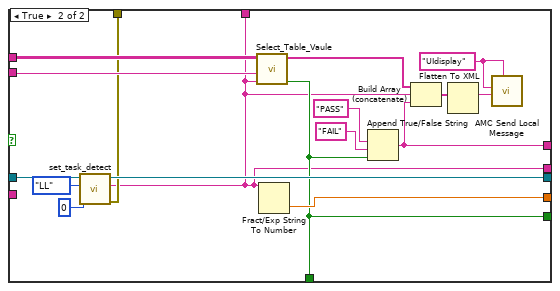
[diagram p19: hidden frame]
diagram:
  n1 = Flush Queue(queue="Message Queue out") -> (queue out=w4:T4)  [unwired: 1 in, 2 out]
  n2 = call "HD_Config.vi"("Step"=enum16{"Initial", "Write", "Read"}."Read") -> ("HD Config out"=w8:T5)  [unwired: 9 in, 1 out]
  n3 = call "AMC Send Local Message.vi"("error in (no error)"="error in (no error)", "Message Name"="LL_Orifice_Size", "Message Queue in"=w4) -> ("error out"=w13:errorcluster, "Message Queue out"=w14:T4)  [unwired: 7 in]
  n4 = while {
    tunnel: w14 -> [w47]
    tunnel: [w43] -> w6
    tunnel: w13 -> [w41]
    tunnel: [w38] -> w5
    shift-right: [w34] -> w10
    shift-left: "?" -> [w35]
    tunnel: w8 -> [w33]
    tunnel: [w29] -> w7
    tunnel: "AllControls In" -> [w22]
    shift-right: [w20] -> w1
    shift-left: "Data in" -> [w21]
    stop <- w23 stop-if-true
    n5 = Wait (ms)(milliseconds to wait=u32 1 ("等待时间（毫秒）")) -> ()  [unwired: 1 out]
    n6 = call "AMC Read Next Message.vi"("error in (no error)"=w41, "timeout (1ms)"=100, "Message Queue in"=w47) -> ("error out"=w40:errorcluster, "Message Value"=w31:string, "Message Name"=w45:string, "Message Queue out"=w46:T4)  [unwired: 1 in, 4 out]
    n7 = case shown="\"LL_Wait_for_X_sec_for_motor_speed_to_stabilise\"" w45 {
      selector: w45 -> [_ w80 w138 w176 w227 w335 w401]
      tunnel: w46 -> [w51 w84 w145 w182 w236 w343 w411]
      tunnel: [w51 w84 w145 w182 w236 w343 w411] -> w44
      tunnel: w40 -> [w50 w83 _ w181 _ w342 _]
      tunnel: [w50 w82 w144 w180 w235 w341 w410] -> w39
      tunnel: [_ w60 w132 _ w216 w327 TRUE] -> w24
      tunnel: w35 -> [w49 w57 w130 w172 w232 w330 w407]
      tunnel: [w49 w57 w130 w172 w231 w339 w406] -> w34
      tunnel: w31 -> [_ w81 w143 w179 w234 w340 w409]
      tunnel: [_ w80 w138 w176 w227 w335 w401] -> w30
      tunnel: w33 -> [_ w67 _ _ _ _ _]
      tunnel: [_ "LL_Motor_On" "LL_Wait_for_X_sec_for_motor_speed_to_stabilise" "LL_get_and_check_DDM_parameter" "LL_Get_and_check_tester_Parameter" w326 w398] -> w32
      tunnel: [_ w53 w133 _ w217 w326 w398] -> w29
      tunnel: w22 -> [_ _ _ _ _ w306 w382]
      tunnel: w21 -> [w48 w56 w129 w168 w214 w318 w394]
      tunnel: [w48 w55 w126 w168 w210 w315 w391] -> w20
      frame "假", Default {
        (unwired) ""
      }
      frame "LL_Orifice_Size" {
        n8 = Unbundle By Name(w56) -> ("Config"=w72:string[][])
        n9 = Unbundle By Name(w67) -> ("NFC.COM"=w73:refnum<visa-resource-name>)
        n10 = call "Index_Config.vi"("Action"="Low_Power_Low_Restriction_Orifice_Size", "config"=w72) -> ("data"=w54:string)  [unwired: 9 in]
        n11 = call "Position_Config.vi"("Step"=enum16{"Initial", "Write", "Read"}."Read") -> ("Position Config out"=w69:T9)  [unwired: 9 in, 1 out]
        n12 = case shown="\"12.7\", Default" w54 {
          tunnel: w69 -> [w88 w90 w92 w94]
          tunnel: [w87 w89 w91 w93] -> w68
          frame "12.7", Default {
            n13 = Unbundle By Name(w88) -> ("Black"=w87:i32)
          }
          frame "13" {
            n14 = Unbundle By Name(w90) -> ("White"=w89:i32)
          }
          frame "30" {
            n15 = Unbundle By Name(w92) -> ("Black1"=w91:i32)
          }
          frame "16" {
            n16 = Unbundle By Name(w94) -> ("White1"=w93:i32)
          }
        }
        n17 = call "IO.vi"("DO DATA"=bool[] [FALSE] ("Writel_IO"), "IO Name"=string[] ["Orifice_fixed_Cylinder"], "IO?"=enum16{"DI", "DO"}."DO") -> ("error out"=w63:errorcluster)  [unwired: 7 in, 1 out]
        n18 = To Long Integer(number=w68) -> (32bit integer=w75:i32)
        n19 = call "Time Delay"("error in (no error)"=w63) -> ("error out"=w62:errorcluster)  [unwired: 10 in]
        n20 = call "LogStatus.vi"("error in (no error)"=w83, "last message"=w81, "message"=w80) -> ("error  out"=w82:errorcluster)  [unwired: 8 in]
        n21 = call "Pulse.vi"("Pulse"=w75) -> ("Pulse"=w76:string)  [unwired: 10 in]
        n22 = call "Motor Visa.vi"("错误输入（无错误）"=w62, "Command"=w76, "VISA资源名称"=w73) -> ("错误输出"=w77:errorcluster, "VISA资源名称输出"=w78:refnum<visa-resource-name>)  [unwired: 6 in, 1 out]
        n23 = call "ABS.vi"() -> ("绝对模式"=w74:string)  [unwired: 11 in]
        n24 = call "Motor Visa.vi"("错误输入（无错误）"=w77, "Command"=w74, "VISA资源名称"=w78) -> ("VISA资源名称输出"=w61:refnum<visa-resource-name>)  [unwired: 6 in, 2 out]
        n25 = while {
          tunnel: w61 -> [w124]
          tunnel: [w109] -> w59
          tunnel: [w103] -> w58
          stop <- w114 stop-if-true
          n26 = call "Get Status.vi"() -> ("Command"=w125:string)  [unwired: 11 in]
          n27 = call "Get Alarm  Error Status.vi"() -> ("AlarmStatus"=w117:string, "ErrorStatus"=w118:string)  [unwired: 10 in]
          n28 = call "Motor Visa.vi"("Command"=w125, "VISA资源名称"=w124) -> ("读取缓冲区"=w123:string, "VISA资源名称输出"=w116:refnum<visa-resource-name>)  [unwired: 7 in, 1 out]
          n29 = Wait (ms)(milliseconds to wait=u32 50 ("等待时间（毫秒）")) -> ()  [unwired: 1 out]
          n30 = call "Motor Visa.vi"("Command"=w118, "VISA资源名称"=w116) -> ("读取缓冲区"=w120:string, "VISA资源名称输出"=w121:refnum<visa-resource-name>)  [unwired: 7 in, 1 out]
          n31 = call "Motor Visa.vi"("Command"=w117, "VISA资源名称"=w121) -> ("读取缓冲区"=w119:string)  [unwired: 7 in, 2 out]
          n32 = call "6-AlarmStatus.vi"("Step"=enum16{"Initial", "Write", "Read"}."Read") -> ("AlarmValue Out"=w107:bool[])  [unwired: 9 in, 1 out]
          n33 = call "Exit.vi"("Step"=enum16{"Initial", "Write", "Read"}."Read" ("step")) -> ("Exit Out"=w105:bool)  [unwired: 9 in, 1 out]
          n34 = call "Stop.vi"("Step"=enum16{"Initial", "Write", "Read"}."Read") -> ("Stop Out"=w104:bool)  [unwired: 9 in, 1 out]
          n35 = call "Alarm and Error Result.vi"("Command"=w119) -> ("Alarm or Error"=w111:bool)  [unwired: 10 in]
          n36 = call "Alarm and Error Result.vi"("Command"=w120) -> ("Alarm or Error"=w110:bool)  [unwired: 10 in]
          n37 = call "Motion Down.vi"("Command"=w123) -> ("Motion Down"=w115:bool)  [unwired: 10 in]
          n38 = Or Array Elements(Boolean array=w107) -> (logical OR=w106:bool)
          n39 = Compound Arithmetic op=OR(w106, w105, w104, w111, w110, w115) -> (w114:bool)
          n40 = Or(x=w111, y=w110) -> (x .or. y?=w109:bool)
          n41 = Compound Arithmetic op=OR(w106, w105, w104) -> (w103:bool)
        }
        n42 = Bundle By Name(cluster=w56, "LL.Restriction Plate Diameter"=w54, "LL_Status.Restriction Plate Diameter"="PASS") -> (w55:T1)
        n43 = case shown="True" w58 {
          tunnel: w61 -> [_ w85]
          frame False {
          }
          frame True {
            n44 = call "Stop Command.vi"() -> ("Stop"=w86:string)  [unwired: 11 in]
            n45 = call "Motor Visa.vi"("Command"=w86, "VISA资源名称"=w85) -> ()  [unwired: 7 in, 3 out]
          }
        }
        n46 = case shown="True" w59 {
          tunnel: [_ "Error" ("Message Name")] -> w53
          frame False {
            n47 = call "IO.vi"("DO DATA"=bool[] [TRUE] ("Writel_IO"), "IO Name"=string[] ["Orifice_fixed_Cylinder"], "IO?"=enum16{"DI", "DO"}."DO") -> ("error out"=w98:errorcluster)  [unwired: 7 in, 1 out]
            n48 = call "Time Delay2"("error in (no error)"=w98) -> ()  [unwired: 10 in, 1 out]
          }
          frame True {
            n49 = call "6-AlarmStatus.vi"("AlarmValue"=TRUE, "AlarmIndex"=AlarmIndex."Motor Error", "Step"=enum16{"Initial", "Write", "Read"}."Write") -> ()  [unwired: 7 in, 2 out]
          }
        }
        n50 = Or(x=w58, y=w59) -> (x .or. y?=w60:bool)
      }
      frame "LL_Motor_On" {
        n51 = Unbundle By Name(w129) -> ("Table"=w137:string[][], "daemon reference"=w142:refnum<k5>, "Config"=w135:string[][])
        n52 = call "Select_Table_Vaule Enable_Disable.vi"("Action"=w138, "Table"=w137) -> ("Enable"=w139:bool)  [unwired: 8 in, 1 out]
        n53 = case shown="True" w139 {
          tunnel: w142 -> [w149 w167]
          tunnel: [TRUE w157] -> _
          tunnel: [w149 w161] -> w127
          tunnel: ["" ("response") w153] -> w131
          tunnel: w138 -> [_ w160]
          tunnel: w137 -> [_ w159]
          tunnel: w135 -> [_ w156]
          tunnel: "Low_Power_Low_Restriction_Drive_Mode" -> [_ w155]
          tunnel: [_ w154] -> w128
          tunnel: [_ w153] -> _
          tunnel: [_ w152] -> _
          tunnel: [_ w151] -> _
          frame False {
          }
          frame True {
            (unwired) "A2" ("Power Mode")
            w166 = "UIdisplay" ("Process (\"\" - local)")
            n54 = call "Index_Config.vi"("Action"=w155, "config"=w156) -> ("data"=w151:string)  [unwired: 9 in]
            n55 = call "drive_motor.vi"("Power Mode"=w151, "daemon reference in"=w167) -> ("error out"=w154:errorcluster, "response"=w153:string, "daemon reference out"=w161:refnum<k5>)  [unwired: 6 in, 1 out]
            n56 = call "Select_Table_Vaule.vi"("Vaule"=w153, "Action"=w160, "Table"=w159) -> ("Result"=w157:bool, "vaule"=w158:string[])  [unwired: 7 in]
            n57 = Append True/False String(1:w157, 2:"FAIL" ("真字符串"), 3:"PASS" ("真字符串")) -> (0:w152:string)  [unwired: 1 in]
            n58 = Build Array (concatenate)(w158, w153, w152) -> (w165:string[])
            n59 = Flatten To XML(anything=w165) -> (xml string=w164:string)
            n60 = call "AMC Send Local Message.vi"("Process (\"\" - local)"=w166, "Message Value"=w164, "Message Name"=w166) -> ()  [unwired: 7 in, 2 out]
          }
        }
        n61 = call <vilib>:"Space Constant.vi"() -> ("String"=w141:string)
        n62 = Concatenate Strings(w138, w141, w131) -> (w140:string)
        n63 = Bundle By Name(cluster=w129, "daemon reference"=w127) -> (w126:T1)
        n64 = call "LogStatus.vi"("error in (no error)"=w128, "last message"=w143, "message"=w140) -> ("error  out"=w144:errorcluster)  [unwired: 8 in]
        n65 = case shown="Error" w128 {
          tunnel: [_ TRUE] -> w132
          tunnel: [_ "Error"] -> w133
          frame No Error {
          }
          frame Error {
          }
        }
      }
      frame "LL_Wait_for_X_sec_for_motor_speed_to_stabilise" {
        (unwired) "10" ("替换字符串(\"\")")
        # "来之Config"
        n66 = Unbundle By Name(w168) -> ("Config"=w174:string[][])
        n67 = call "Index_Config.vi"("Action"="Low_Power_Low_Restriction_Stabilisation_Time" ("替换字符串(\"\")"), "config"=w174) -> ("data"=w171:string)  [unwired: 9 in]
        n68 = Search and Replace String(input string=w176, search string="X" ("搜索字符串"), replace string=w171) -> (result string=w177:string)  [unwired: 5 in, 3 out]
        n69 = Get Date/Time In Seconds() -> (seconds since 1Jan1904=w170:timestamp)
        n70 = Fract/Exp String To Number(string=w171) -> (number=w169:dbl)  [unwired: 3 in, 1 out]
        n71 = while {
          tunnel: w170 -> [w189]
          tunnel: w169 -> [w186]
          tunnel: [w185] -> _
          stop <- w185 stop-if-true
          n72 = Get Date/Time In Seconds() -> (seconds since 1Jan1904=w190:timestamp)
          n73 = Subtract(x=w190, y=w189) -> (x-y=w188:dbl)
          n74 = call "6-AlarmStatus.vi"("Step"=enum16{"Initial", "Write", "Read"}."Read") -> ("AlarmValue Out"=w193:bool[])  [unwired: 9 in, 1 out]
          n75 = Greater Or Equal?(x=w188, y=w186) -> (x >= y?=w187:bool)
          n76 = call "Stop.vi"("Step"=enum16{"Initial", "Write", "Read"}."Read") -> ("Stop Out"=w191:bool)  [unwired: 9 in, 1 out]
          n77 = call "Exit.vi"("Step"=enum16{"Initial", "Write", "Read"}."Read" ("step")) -> ("Exit Out"=w195:bool)  [unwired: 9 in, 1 out]
          n78 = Or Array Elements(Boolean array=w193) -> (logical OR=w192:bool)
          n79 = Compound Arithmetic op=OR(w187, w191, w195, w192) -> (w185:bool)
          n80 = Wait (ms)(milliseconds to wait=u32 1 ("等待时间（毫秒）")) -> ()  [unwired: 1 out]
        }
        n81 = call "LogStatus.vi"("error in (no error)"=w181, "last message"=w179, "message"=w177) -> ("error  out"=w180:errorcluster)  [unwired: 8 in]
      }
      frame "LL_get_and_check_DDM_parameter" {
        n82 = Unbundle By Name(w214) -> ("Table"=w226:string[][], "daemon reference"=w233:refnum<k5>, "Config"=w224:string[][])
        n83 = call "Select_Table_Vaule Enable_Disable.vi"("Action"=w227, "Table"=w226) -> ("Enable"=w225:bool)  [unwired: 8 in, 1 out]
        n84 = case shown="False" w225 {
          tunnel: w233 -> [w242 w268]
          tunnel: [w242 w267] -> w211
          tunnel: [w241 w258] -> w228
          tunnel: w227 -> [_ w264]
          tunnel: w226 -> [_ w269]
          tunnel: w224 -> [_ _]
          tunnel: [_ w253] -> w222
          tunnel: [_ w266] -> w221
          tunnel: [_ w257] -> w213
          tunnel: T7[] ["voltage", "current", "power", "speed", "measured_power", "pressure"] ("Parameter") -> [_ w252]
          tunnel: [w240 w247] -> w212
          tunnel: [w240 w243] -> w203
          frame False {
            w241 = "Skip" ("software string")
            n85 = Initialize Array(w241, 6 ("维数大小")) -> (w240:string[])
          }
          frame True {
            w262 = string[] ["LL_DDM_voltage", "LL_DDM_current", "LL_DDM_power", "LL_DDM_speed", "LL_DDM_measured_power", "LL_DDM_pressure"]
            n86 = for {
              tunnel: [w275] -> w250 mode=indexing
              tunnel: [w274] -> w257
              tunnel: [w270] -> w254 mode=indexing
              tunnel: w252 -> [w272] mode=indexing
              shift-right: [w276] -> w267
              shift-left: w268 -> [w277]
              n87 = Build Array(w272) -> (w271:T7[])
              n88 = call "get_parameter.vi"("Parameter"=w271, "daemon reference in"=w277) -> ("error out"=w274:errorcluster, "response"=w275:string, "values"=w273:dbl[], "daemon reference out"=w276:refnum<k5>)  [unwired: 5 in, 1 out]
              n89 = Index Array(array=w273) -> (element=w270:dbl)  [unwired: 1 in]
            }
            n90 = in-place {
              w282 = 1000.0
              n91 = in-place-array #1(w254, 3, 5) -> (w281:dbl, w278:dbl)
              n92 = Divide(x=w281, y=w282) -> (x/y=w280:dbl)
              n93 = Divide(x=w278, y=w282) -> (x/y=w279:dbl)
              n94 = in-place-array #1(w280, w279) -> (w253:dbl[])  [unwired: 2 out]
            }
            n95 = Array To Spreadsheet String(delimiter (Tab)=",", array=w250, 3:"" ("format string")) -> (spreadsheet string=w251:string)
            n96 = Number To Fractional String(number=w253) -> (F-format string=w247:string[])  [unwired: 3 in]
            n97 = Interleave 1D Arrays(w262, w247) -> (w261:string[])
            n98 = Array To Spreadsheet String(delimiter (Tab)=";" ("格式字符串"), array=w261, 3:"" ("格式字符串")) -> (spreadsheet string=w258:string)
            n99 = Build Array (concatenate)(w264, w262) -> (w265:string[])
            n100 = Build Array (concatenate)(w251, w247) -> (w263:string[])
            n101 = for {
              tunnel: w269 -> [w289]
              tunnel: w263 -> [w287] mode=indexing
              tunnel: w265 -> [w286] mode=indexing
              tunnel: [w285] -> w266 mode=indexing
              tunnel: [w283] -> w244 mode=indexing
              w294 = "UIdisplay" ("Process (\"\" - local)")
              n102 = call "Select_Table_Vaule.vi"("Boolean"=TRUE, "Vaule"=w287, "Action"=w286, "Table"=w289) -> ("Result"=w285:bool, "vaule"=w288:string[])  [unwired: 6 in]
              n103 = Append True/False String(1:w285, 2:"FAIL" ("真字符串"), 3:"PASS" ("真字符串")) -> (0:w283:string)  [unwired: 1 in]
              n104 = Build Array (concatenate)(w288, w287, w283) -> (w293:string[])
              n105 = Flatten To XML(anything=w293) -> (xml string=w292:string)
              n106 = call "AMC Send Local Message.vi"("Process (\"\" - local)"=w294, "Message Value"=w292, "Message Name"=w294) -> ()  [unwired: 7 in, 2 out]
            }
            n107 = Delete From Array(array=w244, length=1 ("长度"), index=0 ("索引")) -> (array with subset deleted=w243:string[])  [unwired: 1 out]
          }
        }
        n108 = call <vilib>:"Space Constant.vi"() -> ("String"=w230:string)
        n109 = Concatenate Strings(w227, w230, w228) -> (w229:string)
        n110 = Index Array(array=w212) -> (element #1=w209:string, element #2=w208:string, element #3=w207:string, element #4=w205:string, element #5=w204:string, element #6=w206:string)  [unwired: 6 in]
        n111 = Delete From Array(array=w221, length=1 ("长度"), index=0 ("索引")) -> (array with subset deleted=w220:bool[])  [unwired: 1 out]
        n112 = Index Array(array=w203) -> (element #1=w202:string, element #2=w201:string, element #3=w200:string, element #4=w198:string, element #5=w199:string, element #6=w197:string)  [unwired: 6 in]
        n113 = Bundle By Name(cluster=w214, "daemon reference"=w211, "LL.LL - DDM Parameter - Voltage"=w209, "LL.LL - DDM Parameter - Current"=w208, "LL.LL - DDM Parameter - Power"=w207, "LL.LL - DDM Parameter - Measured Power"=w204, "LL.LL - DDM Parameter - Speed"=w205, "LL.LL - DDM Parameter - Pressure"=w206, "LL_Status.LL - DDM Parameter - Voltage"=w202, "LL_Status.LL - DDM Parameter - Current"=w201, "LL_Status.LL - DDM Parameter - Power"=w200, "LL_Status.LL - DDM Parameter - Measured Power"=w199, "LL_Status.LL - DDM Parameter - Speed"=w198, "LL_Status.LL - DDM Parameter - Pressure"=w197) -> (w210:T1)
        n114 = call "LogStatus.vi"("error in (no error)"=w213, "last message"=w234, "message"=w229) -> ("error  out"=w235:errorcluster)  [unwired: 8 in]
        n115 = Bundle By Name(cluster=w232, "Task_Detect_Calib.LL.DDM_Parameter"=w222, "Task_Detect_Calib.LL.DDM_Parameter_status"=w220) -> (w231:T3)
        n116 = case shown="Error" w213 {
          tunnel: [_ TRUE] -> w216
          tunnel: [_ "Error"] -> w217
          frame No Error {
          }
          frame Error {
          }
        }
      }
      frame "LL_Get_and_check_tester_Parameter" {
        n117 = Unbundle By Name(w330) -> ("Task_Detect_Calib.LL.DDM_Parameter"=w321:dbl[])
        n118 = Unbundle By Name(w318) -> ("Table"=w320:string[][], "daemon reference"=w319:refnum<k5>)
        n119 = call "Select_Table_Vaule Enable_Disable.vi"("Action"=w335, "Table"=w320) -> ("Enable"=w334:bool)  [unwired: 8 in, 1 out]
        n120 = case shown="False" w334 {
          tunnel: w319 -> [w347 w365]
          tunnel: [w347 w365] -> w316
          tunnel: [w346 w356] -> w336
          tunnel: w335 -> [_ w362]
          tunnel: w320 -> [_ w366]
          tunnel: [_ w353] -> w333
          tunnel: [_ w364] -> w325
          tunnel: w321 -> [_ w354]
          tunnel: [w345 w352] -> w317
          tunnel: [w345 w348] -> w299
          frame False {
            w346 = "Skip" ("software string")
            n121 = Initialize Array(w346, 4 ("维数大小")) -> (w345:string[])
          }
          frame True {
            w355 = string[] ["LL_Tester_Voltage", "LL_Tester_Current", "LL_Tester_Power", "LL_DDM_Real_Power"]
            n122 = call "Task_Detect_Calibration_Calculate_Tester_Parameter.vi"("DDM Parameter"=w354) -> ("Calculate Tester Parameter"=w353:dbl[])  [unwired: 10 in]
            n123 = Number To Fractional String(number=w353) -> (F-format string=w352:string[])  [unwired: 3 in]
            n124 = Interleave 1D Arrays(w355, w352) -> (w359:string[])
            n125 = Array To Spreadsheet String(delimiter (Tab)=";" ("格式字符串"), array=w359, 3:"" ("格式字符串")) -> (spreadsheet string=w356:string)
            n126 = Build Array (concatenate)(w362, w355) -> (w363:string[])
            n127 = Build Array (concatenate)("", w352) -> (w361:string[])
            n128 = for {
              tunnel: w366 -> [w372]
              tunnel: w361 -> [w370] mode=indexing
              tunnel: w363 -> [w369] mode=indexing
              tunnel: [w368] -> w364 mode=indexing
              tunnel: [w367] -> w349 mode=indexing
              w377 = "UIdisplay" ("Process (\"\" - local)")
              n129 = call "Select_Table_Vaule.vi"("Vaule"=w370, "Action"=w369, "Table"=w372) -> ("Result"=w368:bool, "vaule"=w371:string[])  [unwired: 7 in]
              n130 = Append True/False String(1:w368, 2:"FAIL" ("真字符串"), 3:"PASS" ("真字符串")) -> (0:w367:string)  [unwired: 1 in]
              n131 = Build Array (concatenate)(w371, w370, w367) -> (w376:string[])
              n132 = Flatten To XML(anything=w376) -> (xml string=w375:string)
              n133 = call "AMC Send Local Message.vi"("Process (\"\" - local)"=w377, "Message Value"=w375, "Message Name"=w377) -> ()  [unwired: 7 in, 2 out]
            }
            n134 = Delete From Array(array=w349, length=1 ("长度"), index=0 ("索引")) -> (array with subset deleted=w348:string[])  [unwired: 1 out]
          }
        }
        n135 = Unbundle By Name(w330) -> ("Task_Detect_Calib.LL.DDM_Parameter_status"=w329:bool[])
        n136 = call <vilib>:"Space Constant.vi"() -> ("String"=w338:string)
        n137 = Concatenate Strings(w335, w338, w336) -> (w337:string)
        n138 = Unbundle By Name(w306) -> ("MES bool"=w311:refnum<vi>)
        n139 = call "HD_Config.vi"("Step"=enum16{"Initial", "Write", "Read"}."Read") -> ("HD Config out"=w310:T5)  [unwired: 9 in, 1 out]
        n140 = Unbundle By Name(w310) -> ("Fail_resume_mode"=w312:bool)
        n141 = property class="Bool (严格)"(reference=w311) -> ("Value"=w313:bool)  [unwired: 1 in, 2 out]
        n142 = Index Array(array=w299) -> (element #1=w298:string, element #2=w297:string, element #3=w296:string, element #4=w295:string)  [unwired: 4 in]
        n143 = Index Array(array=w317) -> (element #1=w303:string, element #2=w302:string, element #3=w301:string, element #4=w300:string)  [unwired: 4 in]
        n144 = Delete From Array(array=w325, length=1 ("长度"), index=0 ("索引")) -> (array with subset deleted=w324:bool[])  [unwired: 1 out]
        n145 = Not(x=w313) -> (.not. x?=w314:bool)
        n146 = Build Array (concatenate)(w329, w324) -> (w328:bool[])
        n147 = Or(x=w312, y=w314) -> (x .or. y?=w309:bool)
        n148 = And Array Elements(Boolean array=w328) -> (logical AND=w304:bool)
        n149 = Bundle By Name(cluster=w318, "daemon reference"=w316, "LL.LL - Tester Parameter - Voltage"=w303, "LL.LL - Tester Parameter - Current"=w302, "LL.LL - Tester Parameter - Power"=w301, "LL.LL - DDM Real Power"=w300, "LL_Status.LL - Tester Parameter - Voltage"=w298, "LL_Status.LL - Tester Parameter - Current"=w297, "LL_Status.LL - Tester Parameter - Power"=w296, "LL_Status.LL - DDM Real Power"=w295) -> (w315:T1)
        n150 = Select(t=TRUE, s=w309, f=w304) -> (s? t:f=w305:bool)
        n151 = Bundle By Name(cluster=w330, "Task_Detect_Calib.LL.Get_Tester_Parameter"=w333, "Task_Detect_Calib.LL.Get_Tester_Parameter_status"=w324) -> (w339:T3)
        n152 = call "LogStatus.vi"("error in (no error)"=w342, "last message"=w340, "message"=w337) -> ("error  out"=w341:errorcluster)  [unwired: 8 in]
        n153 = Select(t="Calibrate_task_detect-LL(A)", s=w305, f="Finalization_NG_unit") -> (s? t:f=w326:string)
        n154 = Not(x=w305) -> (.not. x?=w327:bool)
      }
      frame "Calibrate_task_detect-LL(A)" {
        n155 = Unbundle By Name(w394) -> ("Table"=w400:string[][], "daemon reference"=w408:refnum<k5>, "Config"=w399:string[][])
        n156 = call "Select_Table_Vaule Enable_Disable.vi"("Action"=w401, "Table"=w400) -> ("Enable"=w402:bool)  [unwired: 8 in, 1 out]
        n157 = case shown="False" w402 {
          tunnel: w408 -> [w418 w436]
          tunnel: [TRUE w422] -> w381
          tunnel: [w418 w430] -> w392
          tunnel: [w417 w421] -> w403
          tunnel: w401 -> [_ w429]
          tunnel: w400 -> [_ w428]
          tunnel: w399 -> [_ _]
          tunnel: [_ w424] -> w396
          tunnel: [_ w423] -> w393
          tunnel: [_ w422] -> w395
          tunnel: [w417 w421] -> w379
          tunnel: [w417 w420] -> w378
          frame False {
            w417 = "Skip" ("response")
          }
          frame True {
            w435 = "UIdisplay" ("Process (\"\" - local)")
            n158 = call "set_task_detect.vi"("Action"=0, "Test Point"=task_detect_test_point."LL", "daemon reference in"=w436) -> ("error out"=w423:errorcluster, "response"=w421:string, "daemon reference out"=w430:refnum<k5>)  [unwired: 5 in, 1 out]
            n159 = call "Select_Table_Vaule.vi"("Vaule"=w421, "Action"=w429, "Table"=w428) -> ("Result"=w422:bool, "vaule"=w427:string[])  [unwired: 7 in]
            n160 = Fract/Exp String To Number(string=w421) -> (number=w424:dbl)  [unwired: 3 in, 1 out]
            n161 = Append True/False String(1:w422, 2:"FAIL" ("真字符串"), 3:"PASS" ("真字符串")) -> (0:w420:string)  [unwired: 1 in]
            n162 = Build Array (concatenate)(w427, w421, w420) -> (w434:string[])
            n163 = Flatten To XML(anything=w434) -> (xml string=w433:string)
            n164 = call "AMC Send Local Message.vi"("Process (\"\" - local)"=w435, "Message Value"=w433, "Message Name"=w435) -> ()  [unwired: 7 in, 2 out]
          }
        }
        n165 = call <vilib>:"Space Constant.vi"() -> ("String"=w405:string)
        n166 = Concatenate Strings(w401, w405, w403) -> (w404:string)
        n167 = Unbundle By Name(w382) -> ("MES bool"=w387:refnum<vi>)
        n168 = call "HD_Config.vi"("Step"=enum16{"Initial", "Write", "Read"}."Read") -> ("HD Config out"=w386:T5)  [unwired: 9 in, 1 out]
        n169 = Unbundle By Name(w386) -> ("Fail_resume_mode"=w388:bool)
        n170 = property class="Bool (严格)"(reference=w387) -> ("Value"=w389:bool)  [unwired: 1 in, 2 out]
        n171 = Not(x=w389) -> (.not. x?=w390:bool)
        n172 = Or(x=w388, y=w390) -> (x .or. y?=w385:bool)
        n173 = Select(t=TRUE, s=w385, f=w381) -> (s? t:f=w380:bool)
        n174 = Bundle By Name(cluster=w394, "LL_Status.LL - Calibrate Task Detect LL"=w378, "LL.LL - Calibrate Task Detect LL"=w379, "daemon reference"=w392) -> (w391:T1)
        n175 = case shown="No Error" w393 {
          tunnel: [w413 "Error"] -> w398
          tunnel: w380 -> [w412 _]
          frame No Error {
            n176 = Select(t="HL_Restriction", s=w412, f="Finalization_NG_unit") -> (s? t:f=w413:string)
          }
          frame Error {
          }
        }
        n177 = Bundle By Name(cluster=w407, "Task_Detect_Calib.LL.Set_task_detect_A"=w396, "Task_Detect_Calib.LL.Set_task_detect_A_Status"=w395) -> (w406:T3)
        n178 = call "LogStatus.vi"("error in (no error)"=w393, "last message"=w409, "message"=w404) -> ("error  out"=w410:errorcluster)  [unwired: 8 in]
      }
    }
    n179 = call "6-AlarmStatus.vi"("Step"=enum16{"Initial", "Write", "Read"}."Read") -> ("AlarmValue Out"=w18:bool[])  [unwired: 9 in, 1 out]
    n180 = call "Stop.vi"("Step"=enum16{"Initial", "Write", "Read"}."Read") -> ("Stop Out"=w26:bool)  [unwired: 9 in, 1 out]
    n181 = call "Exit.vi"("Step"=enum16{"Initial", "Write", "Read"}."Read" ("step")) -> ("Exit Out"=w25:bool)  [unwired: 9 in, 1 out]
    n182 = Or Array Elements(Boolean array=w18) -> (logical OR=w17:bool)
    n183 = Compound Arithmetic op=OR(w24, w26, w25, w17) -> (w23:bool)
    n184 = call "AMC Run Step.vi"("Message Queue In"=w44, "Message Name"=w32, "Message Value"=w30, "error in (no error)"=w39, "Mli/Sig"=FALSE) -> ("Message Queue Out"=w43:T4, "error out"=w38:errorcluster)  [unwired: 13 in]
  }
  "Message Queue Out" <- w6
  "error out" <- w5
  "Data" <- w10
  "Flow" <- w7
  "Data out" <- w1
